vi "fit function - einstein.vi"(3 "output control":T1, 4 "data":T2, 5 "X":dbl[](array[numeric]), 6 "a":dbl[](array[numeric])) -> (0 "error out":errorcluster, 1 "f'(X,a)":dbl[][](array[numeric]), 2 "f(X,a)":dbl[](array[numeric]))   [LabVIEW 2021]
doc: "This template is the starting point for creating a model function to be passed to the Nonlinear Curve Fit.vi."
uses:
  <vilib>/gmath/NumericalOptimization/objective function data.ctl
  <vilib>/gmath/NumericalOptimization/LM_output select.ctl
  <vilib>/gmath/NI_Gmath.lvlib
panel:
  in  "fit":enum16{"other", "3par", "5par"}(ring)=enum."3par"
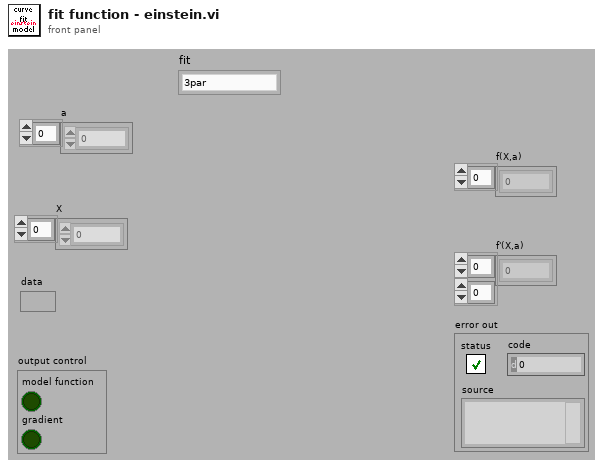
[diagram p1: front panel]
types:
  T1 = typedef "NI_Gmath.lvlib/LM_output select.ctl" = cluster{"model function":bool, "gradient":bool}
  T2 = typedef "NI_Gmath.lvlib/objective function data.ctl" = variant
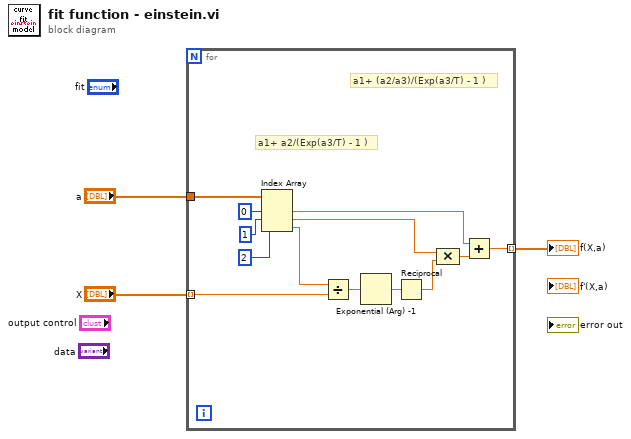
[diagram p0: block diagram]
diagram:
  n1 = for {
    tunnel: "a" -> [w16]
    tunnel: "X" -> [w14] mode=indexing
    tunnel: [w15] -> w1 mode=indexing
    # "a1+ (a2/a3)/(Exp(a3/T) - 1 )"
    # "a1+ a2/(Exp(a3/T) - 1 )"
    n2 = Index Array(array=w16, index #1=0 ("index"), index #2=1 ("index"), index #3=2 ("index")) -> (element #1=w6:dbl, element #2=w9:dbl, element #3=w4:dbl)
    n3 = Divide(x=w4, y=w14) -> (x/y=w5:dbl)
    n4 = Exponential (Arg) -1(1:w5) -> (0:w10:dbl)
    n5 = Reciprocal(x=w10) -> (1/x=w8:dbl)
    n6 = Compound Arithmetic op=MULTIPLY(w9, w8) -> (w7:dbl)
    n7 = Add(x=w6, y=w7) -> (x+y=w15:dbl)
  }
  "f(X,a)" <- w1
